vi "BRig_RT_storeData__1D_dbl.vi"(10 "Array":dbl[](array[numeric]), 11 "input_filename":string) -> ()   [LabVIEW 2014]
uses:
  <vilib>/Utility/file.llb/Write To Spreadsheet File (DBL).vi
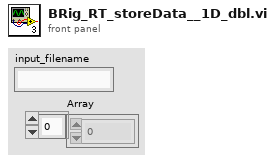
[diagram p1: front panel]
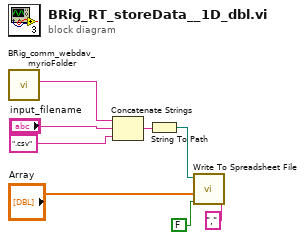
[diagram p0: block diagram]
diagram:
  n1 = call "BRig_comm_webdav_myrioFolder.vi"() -> ("output_myrioFolder"=w5:string)  [unwired: 11 in]
  n2 = Concatenate Strings(w5, "input_filename", ".csv" ("string")) -> (w3:string)
  n3 = String To Path(string=w3) -> (path=w2:path)
  n4 = call-poly <vilib>:"Write To Spreadsheet File.vi"("delimiter (\\t)"="," ("delimiter (\\t)"), "append to file? (new file:F)"=FALSE, "1D data"="Array", "file path (dialog if empty)"=w2) -> ()  [unwired: 4 in, 1 out]
